vi "Diode_Check.vi"(6 "Stim.On?":bool, 7 "Timer Handle":T1, 8 "error in (no error)":errorcluster, 9 "Diode Currents":waveform(dbl)[](array[waveform])=[{"t0"=timestamp(3845890993.434256 s since 1904-01-01), "dt"=1.0, "Y"=[0.0]}, {"t0"=timestamp(3845890993.434256 s since 1904-01-01), "dt"=1.0, "Y"=[0.0]}], 10 "TED Status":T2[](array[typedef])=[{"Output"=TRUE, "SetPoint"=0.0, "Temperature"=0.0, "Current"=0.0, "Voltage"=0.0, "CableTrip"=FALSE, "TransducerTrip"=FALSE, "OverTemp"=FALSE}, {"Output"=TRUE, "SetPoint"=0.0, "Temperature"=0.0, "Current"=0.0, "Voltage"=0.0, "CableTrip"=FALSE, "TransducerTrip"=FALSE, "OverTemp"=FALSE}], 11 "Diode Test Options":T3={"Temp.Tol"=0.1, "Max IDark"=[0.1, 1e-07], "Min ILight"=[0.15, 1e-06], "Min TEC \nCurrent"=0.2, "Max TEC \nCurrent"=1.0}) -> (0 "error out":errorcluster, 1 "TEC Faults":bool[](array[boolean])=[TRUE, TRUE], 5 "Timer Handle Out":T1)   [LabVIEW 2025]
doc: "Use this template to build a VI to use as a subVI."
uses:
  controls/Diode Test Options.ctl
  controls/TED4015 Status.ctl
  <vilib>/NI/Timer/Typedefs/Session Handle.ctl
  <vilib>/NI/Timer/Timer Session.lvclass
  <userlib>/_OpenG.lib/comparison/comparison.llb/Boolean Changed__ogtk.vi
  <userlib>/_OpenG.lib/comparison/comparison.llb/openg_comparison__ogtk.lvlib
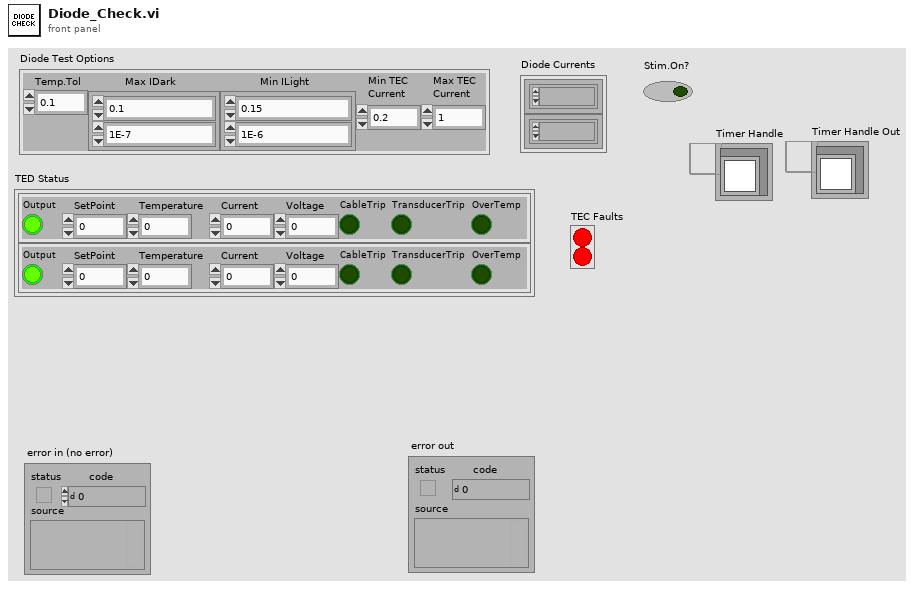
[diagram p1: front panel]
types:
  T1 = typedef "Timer Session.lvclass/Session Handle.ctl" = refnum<data-value>
  T2 = typedef "TED4015 Status.ctl" = cluster{"Output":bool, "SetPoint":dbl, "Temperature":dbl, "Current":dbl, "Voltage":dbl, "CableTrip":bool, "TransducerTrip":bool, "OverTemp":bool}
  T3 = typedef "Diode Test Options.ctl" = cluster{"Temp.Tol":dbl, "Max IDark":dbl[], "Min ILight":dbl[], "Min TEC \nCurrent":dbl, "Max TEC \nCurrent":dbl}
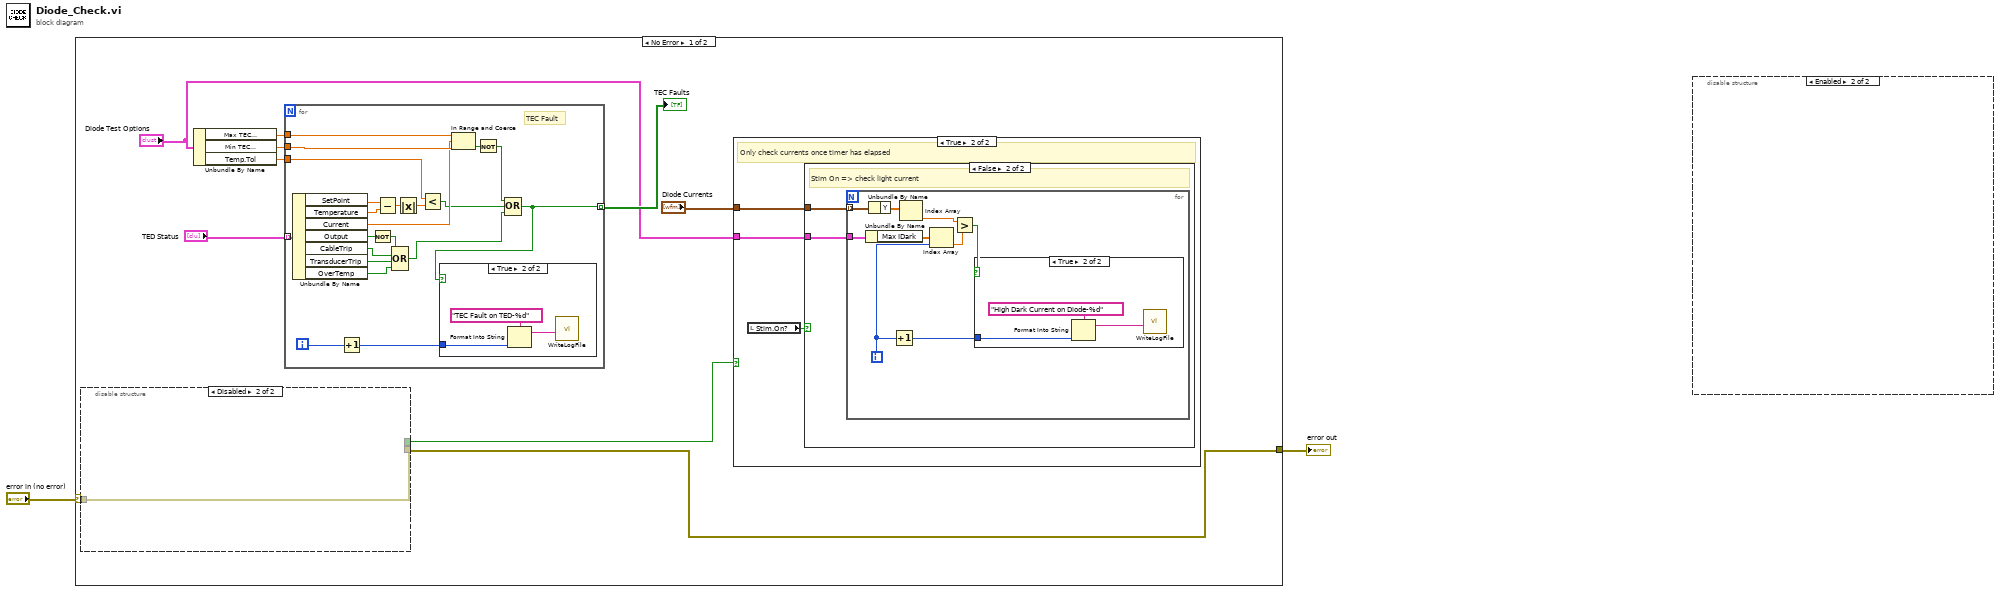
[diagram p0: block diagram]
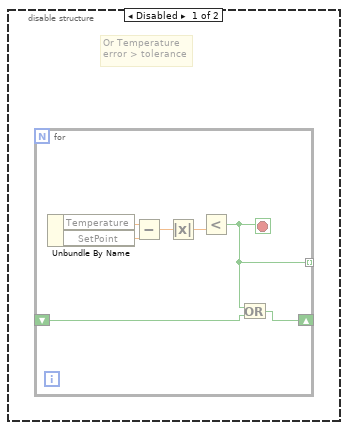
[diagram p2: hidden frame]
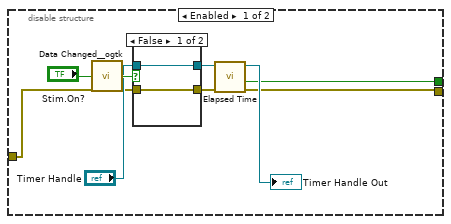
[diagram p3: hidden frame]
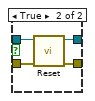
[diagram p4: hidden frame]
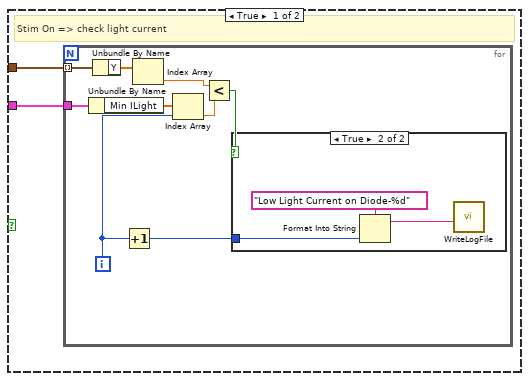
[diagram p6: hidden frame]
diagram:
  n1 = case shown="No Error" "error in (no error)" {
    selector: "error in (no error)" -> [w12 w84]
    tunnel: [w3 w84] -> w1
    frame No Error {
      n2 = disable-structure shown="Disabled" {
        disable-tunnel: w12 -> [w18 w28]
        disable-tunnel: [w14 w28] -> w3
        disable-tunnel: [w13 _] -> w6
        frame Enabled {
          n3 = call-poly <userlib>:"Data Changed__ogtk.vi"("Boolean"="Stim.On?") -> ("Changed"=w20:bool)
          n4 = case shown="False" w20 {
            tunnel: "Timer Handle" -> [w23 w27]
            tunnel: w18 -> [w22 w26]
            tunnel: [w22 w25] -> w17
            tunnel: [w23 w24] -> w16
            frame False {
            }
            frame True {
              n5 = call <vilib>:"Reset.vi"("Error In"=w26, "Timer Handle"=w27) -> ("Error Out"=w25:errorcluster, "Timer Handle"=w24:T1)  [unwired: 8 in]
            }
          }
          n6 = call <vilib>:"Elapsed Time.vi"("Error In"=w17, "Timer Handle"=w16) -> ("Error Out"=w14:errorcluster, "Time Elapsed"=w13:bool, "Timer Handle"=→"Timer Handle Out":T1)  [unwired: 6 in, 1 out]
        }
        frame Disabled {
        }
      }
      n7 = Unbundle By Name("Diode Test Options") -> ("Max TEC \nCurrent"=w11:dbl, "Min TEC \nCurrent"=w10:dbl, "Temp.Tol"=w4:dbl)
      n8 = for {
        tunnel: w11 -> [w80]
        tunnel: w10 -> [w79]
        tunnel: [w61] -> w8 mode=indexing
        tunnel: "TED Status" -> [w76] mode=indexing
        tunnel: w4 -> [w64]
        i -> [w62]
        # "TEC Fault"
        n9 = Unbundle By Name(w76) -> ("SetPoint"=w68:dbl, "Temperature"=w67:dbl, "Current"=w69:dbl, "Output"=w77:bool, "CableTrip"=w75:bool, "TransducerTrip"=w74:bool, "OverTemp"=w73:bool)
        n10 = Increment(x=w62) -> (x+1=w60:i32)
        n11 = Not(x=w77) -> (.not. x?=w72:bool)
        n12 = Subtract(x=w68, y=w67) -> (x-y=w66:dbl)
        n13 = Compound Arithmetic op=OR(w72, w75, w74, w73) -> (w70:bool)
        n14 = Absolute Value(x=w66) -> (abs(x)=w65:dbl)
        n15 = Less?(x=w64, y=w65) -> (x < y?=w63:bool)
        n16 = In Range and Coerce(upper limit=w80, x=w69, lower limit=w79) -> (In Range?=w71:bool)  [unwired: 1 out]
        n17 = Not(x=w71) -> (.not. x?=w78:bool)
        n18 = Compound Arithmetic op=OR(w78, w63, w70) -> (w61:bool)
        n19 = case shown="True" w61 {
          tunnel: w60 -> [_ w82]
          frame False {
          }
          frame True {
            n20 = Format Into String(format string="TEC Fault on TED-%d", w82) -> (resulting string=w81:string)  [unwired: 2 in, 1 out]
            n21 = call "WriteLogFile.vi"("Message"=w81) -> ()  [unwired: 10 in, 1 out]
          }
        }
      }
      "TEC Faults" <- w8
      n22 = case shown="True" w6 {
        tunnel: "Diode Currents" -> [_ w31]
        tunnel: "Diode Test Options" -> [_ w29]
        frame False {
        }
        frame True {
          # "Only check currents once timer has elapsed"
          n23 = local read "Stim.On?"() -> (w30:bool)
          n24 = case shown="False" w30 {
            tunnel: w31 -> [w33 w47]
            tunnel: w29 -> [w32 w46]
            frame True {
              # "Stim On => check light current"
              n25 = for {
                tunnel: w33 -> [w42] mode=indexing
                tunnel: w32 -> [w39]
                i -> [w35]
                n26 = Unbundle By Name(w39) -> ("Min ILight"=w38:dbl[])
                n27 = Unbundle By Name(w42) -> ("Y"=w41:dbl[])
                n28 = Increment(x=w35) -> (x+1=w34:i32)
                n29 = Index Array(array=w41) -> (element=w40:dbl)  [unwired: 1 in]
                n30 = Index Array(array=w38, index=w35) -> (element=w37:dbl)
                n31 = Less?(x=w40, y=w37) -> (x < y?=w36:bool)
                n32 = case shown="True" w36 {
                  tunnel: w34 -> [_ w44]
                  frame False {
                  }
                  frame True {
                    n33 = Format Into String(format string="Low Light Current on Diode-%d", w44) -> (resulting string=w43:string)  [unwired: 2 in, 1 out]
                    n34 = call "WriteLogFile.vi"("Message"=w43) -> ()  [unwired: 10 in, 1 out]
                  }
                }
              }
            }
            frame False {
              # "Stim On => check light current"
              n35 = for {
                tunnel: w47 -> [w56] mode=indexing
                tunnel: w46 -> [w53]
                i -> [w49]
                n36 = Unbundle By Name(w53) -> ("Max IDark"=w52:dbl[])
                n37 = Unbundle By Name(w56) -> ("Y"=w55:dbl[])
                n38 = Increment(x=w49) -> (x+1=w48:i32)
                n39 = Index Array(array=w55) -> (element=w54:dbl)  [unwired: 1 in]
                n40 = Index Array(array=w52, index=w49) -> (element=w51:dbl)
                n41 = Greater?(x=w54, y=w51) -> (0:w50:bool)
                n42 = case shown="True" w50 {
                  tunnel: w48 -> [_ w58]
                  frame False {
                  }
                  frame True {
                    n43 = Format Into String(format string="High Dark Current on Diode-%d", w58) -> (resulting string=w57:string)  [unwired: 2 in, 1 out]
                    n44 = call "WriteLogFile.vi"("Message"=w57) -> ()  [unwired: 10 in, 1 out]
                  }
                }
              }
            }
          }
        }
      }
    }
    frame Error {
    }
  }
  "error out" <- w1
  n45 = disable-structure shown="Enabled" {
    frame Disabled {
      # "Or Temperature\nerror > tolerance"
      n46 = for {
        shift-right: [w86] -> _
        shift-left: _ -> [w87]
        tunnel: [w85] -> _ mode=indexing
        stop <- w85 stop-if-true
        n47 = Unbundle By Name() -> ("Temperature"=w90:dbl, "SetPoint"=w89:dbl)  [unwired: 1 in]
        n48 = Subtract(x=w90, y=w89) -> (x-y=w91:dbl)
        n49 = Absolute Value(x=w91) -> (abs(x)=w88:dbl)
        n50 = Less?(y=w88) -> (x < y?=w85:bool)  [unwired: 1 in]
        n51 = Or(x=w85, y=w87) -> (x .or. y?=w86:bool)
      }
    }
    frame Enabled {
    }
  }
